vi "Skaluj wartosc enkodera FVG.vi"(7 "Akcja (GET)":T1, 8 "error in (no error)":errorcluster, 10 "Impulsy In":waveform(dbl)[](array[waveform]), 11 "Skala":dbl) -> (0 "error out":errorcluster, 2 "Impulsy Out":waveform(dbl)[](array[waveform]))   [LabVIEW 2013]
doc: "Skaluje wartości odczytane z enkodera\nza pomocą współczynnika skali wyliczonego przez wzorcowanie"
uses:
  Kontrolki/FVGs/FVG akcje podstawowa.ctl
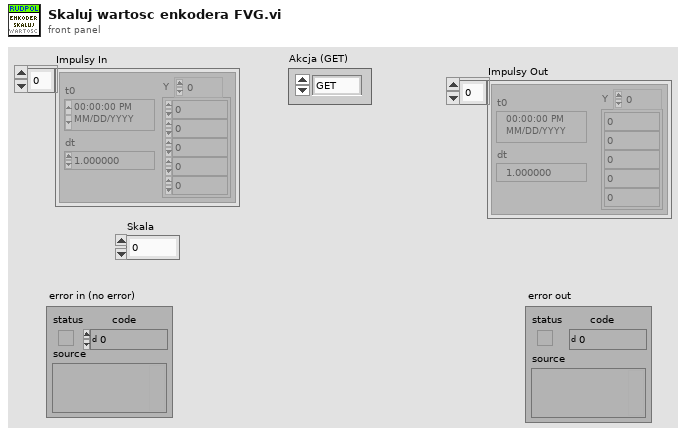
[diagram p1: front panel]
types:
  T1 = typedef "FVG akcje podstawowa.ctl" = enum16{"GET", "SET"}
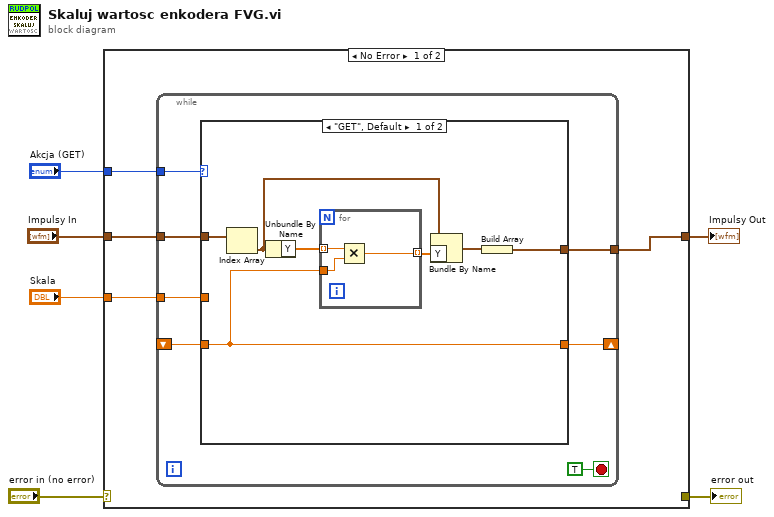
[diagram p0: block diagram]
diagram:
  n1 = case shown="No Error" "error in (no error)" {
    selector: "error in (no error)" -> [_ w31]
    tunnel: [_ w31] -> w5
    tunnel: "Akcja (GET)" -> [w10 _]
    tunnel: "Impulsy In" -> [w9 w30]
    tunnel: "Skala" -> [w8 _]
    tunnel: [w7 w30] -> w1
    frame No Error {
      n2 = while {
        tunnel: w10 -> [w17]
        tunnel: w9 -> [w16]
        tunnel: w8 -> [w15]
        shift-right: [w13] -> _
        shift-left: _ -> [w12]
        tunnel: [w11] -> w7
        stop <- TRUE ("stop") stop-if-true
        n3 = case shown="\"GET\", Default" w17 {
          tunnel: w16 -> [w24 w28]
          tunnel: w15 -> [_ w29]
          tunnel: [w22 w29] -> w13
          tunnel: w12 -> [w22 _]
          tunnel: [w18 w28] -> w11
          frame "GET", Default {
            n4 = Index Array(array=w24) -> (element=w20:waveform(dbl))  [unwired: 1 in]
            n5 = Unbundle By Name(w20) -> ("Y"=w23:dbl[])
            n6 = for {
              tunnel: w23 -> [w27] mode=indexing
              tunnel: w22 -> [w26]
              tunnel: [w25] -> w21 mode=indexing
              n7 = Multiply(x=w27, y=w26) -> (x*y=w25:dbl)
            }
            n8 = Bundle By Name(cluster=w20, "Y"=w21) -> (w19:waveform(dbl))
            n9 = Build Array(w19) -> (w18:waveform(dbl)[])
          }
          frame "SET" {
          }
        }
      }
    }
    frame Error {
    }
  }
  "error out" <- w5
  "Impulsy Out" <- w1
